vi "Agilent DMM Initialize.vi"(8 "error in (no error)":errorcluster, 11 "Configuration":T2={"BusType"=enum."GPIB", "GPIB Bus"=0, "GPIB Address"=16, "IP"=0, "COM"=1, "Baud Rate"=enum."9600"}) -> (0 "error out":errorcluster {"code" format="%.0x"}, 3 "VISA Resource Name":refnum<visa-resource-name>, 5 "Agilent DMM":T1)   [LabVIEW 2011]
uses:
  TypeDefs/Agilent DMM Configuration.ctl
  TypeDefs/Agilent DMM Instrument Info.ctl
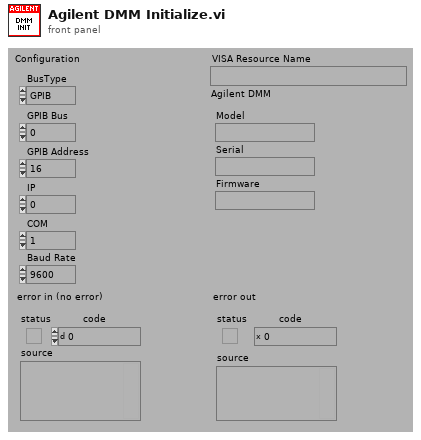
[diagram p1: front panel]
types:
  T1 = typedef "Agilent DMM Instrument Info.ctl" = cluster{"Model":string, "Serial":string, "Firmware":string}
  T2 = typedef "Agilent DMM Configuration.ctl" = cluster{"BusType":enum32{"GPIB", "LAN/IP", "Serial"}, "GPIB Bus":i32, "GPIB Address":i32, "IP":u32, "COM":i32, "Baud Rate":enum16{"300", "600", "1200", "2400", "4800", "9600"}}
  T3 = enum16{"300", "600", "1200", "2400", "4800", "9600"}
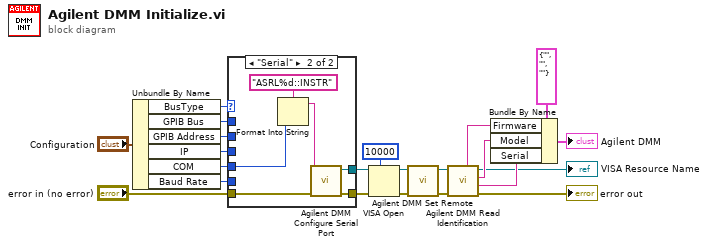
[diagram p0: block diagram]
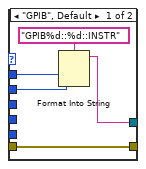
[diagram p2: hidden frame]
diagram:
  n1 = Unbundle By Name("Configuration") -> ("BusType"=w21:enum32{"GPIB", "LAN/IP", "Serial"}, "GPIB Bus"=w20:i32, "GPIB Address"=w19:i32, "IP"=w18:u32, "COM"=w17:i32, "Baud Rate"=w15:T3)
  n2 = case shown="\"Serial\"" w21 {
    tunnel: "error in (no error)" -> [w24 w30]
    tunnel: w20 -> [w27 _]
    tunnel: w19 -> [w26 _]
    tunnel: w18 -> [_ _]
    tunnel: w17 -> [_ w32]
    tunnel: w15 -> [_ _]
    tunnel: [w24 w29] -> w6
    tunnel: [w23 w31] -> w5
    frame "GPIB", Default {
      n3 = Format Into String(format string="GPIB%d::%d::INSTR", w27, w26) -> (resulting string=w23:string)  [unwired: 2 in, 1 out]
    }
    frame "Serial" {
      n4 = Format Into String(format string="ASRL%d::INSTR", w32) -> (resulting string=w28:string)  [unwired: 2 in, 1 out]
      n5 = call "Agilent DMM Configure Serial Port.vi"("error in (no error)"=w30, "VISA Resource Name"=w28) -> ("error out"=w29:errorcluster, "dup VISA Resource Name"=w31:refnum<visa-resource-name>)  [unwired: 8 out]
    }
  }
  n6 = VISA Open(timeout (0)=u32 10000 ("VISA Open timeout (0)"), error in (no error)=w6, VISA resource name=w5) -> (VISA resource name=w1:refnum<visa-resource-name>, error out=w2:errorcluster)  [unwired: 2 out]
  n7 = call "Agilent DMM Set Remote.vi"("error in (no error)"=w2, "VISA Resource Name"=w1) -> ("error out"=w4:errorcluster, "dup VISA Resource Name"=w3:refnum<visa-resource-name>)  [unwired: 8 out]
  n8 = call "Agilent DMM Read Identification.vi"("error in (no error)"=w4, "VISA Resource Name"=w3) -> ("error out"=→"error out":errorcluster, "Serial Number"=w13:string, "Model"=w12:string, "dup VISA Resource Name"=→"VISA Resource Name":refnum<visa-resource-name>, "Firmware"=w14:string)  [unwired: 5 out]
  n9 = Bundle By Name(cluster=T1 {"Model"="", "Serial"="", "Firmware"=""} ("Agilent VNA"), "Firmware"=w14, "Model"=w12, "Serial"=w13) -> (→"Agilent DMM":T1)
